vi "Task4....vi"() -> ()   [LabVIEW 2014, in "Diaz_Excercise_3.lvrbt"]
uses:
  Diaz_Excercise_3.lvrbt
panel:
  out "Waveform Graph":dbl[][](graph)
  out "XY Graph":cluster{"X":dbl, "Y":dbl}[](graph)
  out "sweep chart":cluster{dbl, dbl}(graph)
  out "scope chart":cluster{dbl, dbl}(graph)
  out "Strip chart":cluster{dbl, dbl}(graph)
  out "moving average":dbl
  out "random number":dbl
  in  "stop":bool
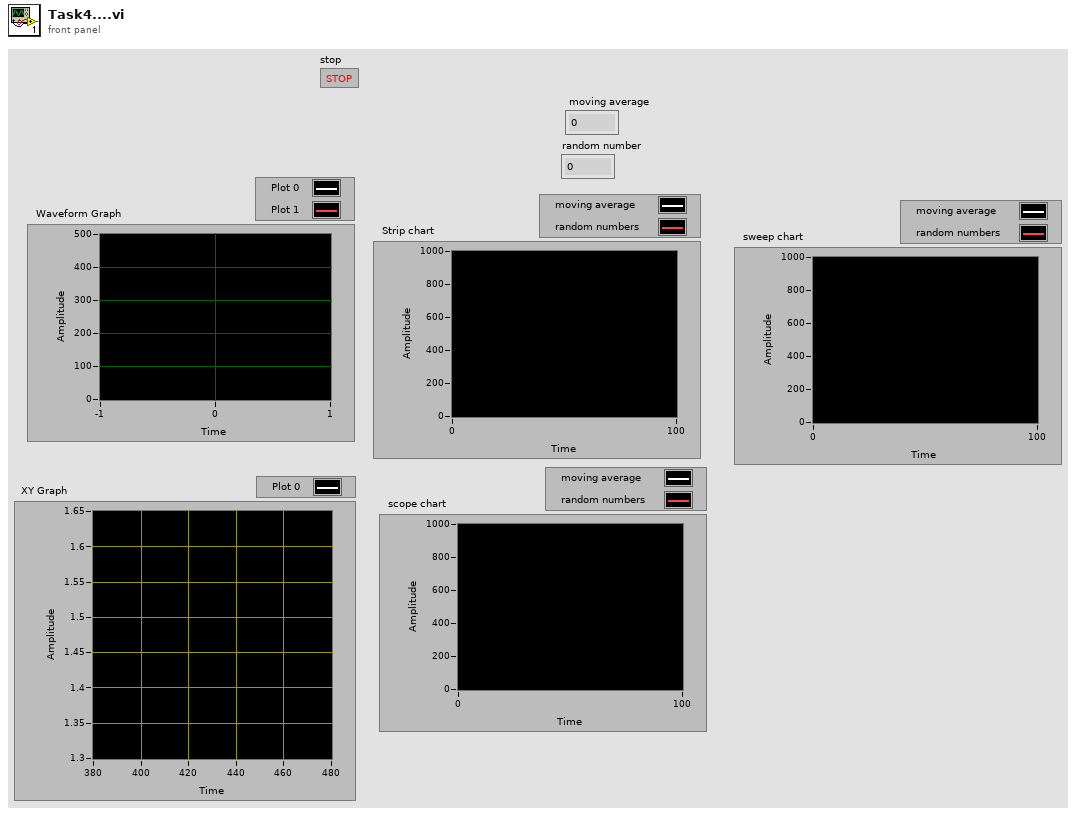
[diagram p1: front panel]
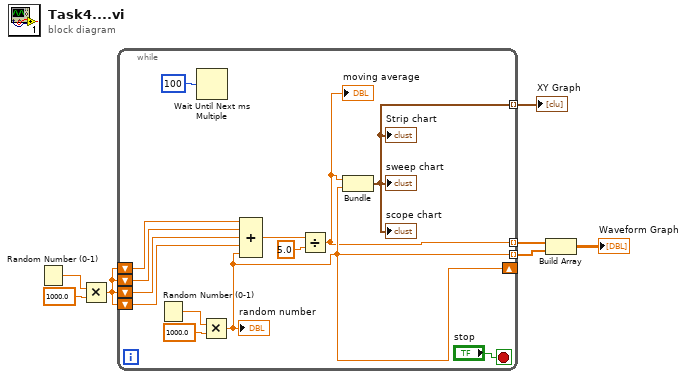
[diagram p0: block diagram]
diagram:
  n1 = Random Number (0-1)() -> (number: 0 to 1=w7:dbl)
  n2 = Multiply(x=w7, y=1000.0) -> (x*y=w5:dbl)
  n3 = while {
    shift-right: [w9] -> _
    shift-left: w5 -> [w15]
    shift-left: w5 -> [w14]
    shift-left: w5 -> [w13]
    shift-left: w5 -> [w12]
    tunnel: [w8] -> w4 mode=indexing
    tunnel: [w9] -> w3 mode=indexing
    tunnel: [w10] -> w2 mode=indexing
    stop <- "stop" stop-if-true
    n4 = Random Number (0-1)() -> (number: 0 to 1=w18:dbl)
    n5 = Wait Until Next ms Multiple(millisecond multiple=u32 100) -> ()  [unwired: 1 out]
    n6 = Multiply(x=w18, y=1000.0) -> (x*y=w9:dbl)
    "random number" <- w9
    n7 = Compound Arithmetic op=ADD(w15, w14, w13, w12, w9) -> (w11:dbl)
    n8 = Divide(x=w11, y=5.0) -> (x/y=w8:dbl)
    "moving average" <- w8
    n9 = Bundle(w8, w9) -> (w10:cluster{dbl, dbl})  [unwired: 1 in]
    "Strip chart" <- w10
    "sweep chart" <- w10
    "scope chart" <- w10
  }
  "XY Graph" <- w2
  n10 = Build Array(w4, w3) -> (→"Waveform Graph":dbl[][])
